vi "Goods subiv.vi"(8 "Status":T2 {"Status - camera" scale=0.0..10.0; "Status - computer" scale=0.0..10.0; "Status - TV" scale=0.0..10.0; "Status - kettle" scale=0.0..10.0; "Status -  microwave" scale=0.0..10.0; "Status - vacuum cleaner" scale=0.0..10.0; "Status - Fridge" scale=0.0..10.0; "Status - washing machine" scale=0.0..10.0}, 9 "Order":T1) -> (2 "avalibity":bool)   [LabVIEW 2020]
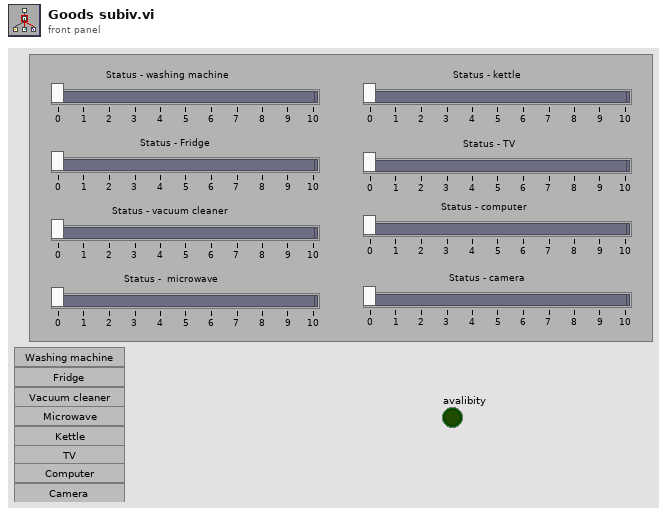
[diagram p1: front panel]
types:
  T1 = cluster{"Washing machine":bool, "Fridge":bool, "Vacuum cleaner":bool, "Microwave":bool, "Kettle":bool, "TV":bool, "Computer":bool, "Camera":bool}
  T2 = cluster{"Status - washing machine":u32, "Status - Fridge":u32, "Status - vacuum cleaner":u32, "Status -  microwave":u32, "Status - kettle":u32, "Status - TV":u32, "Status - computer":u32, "Status - camera":u32}
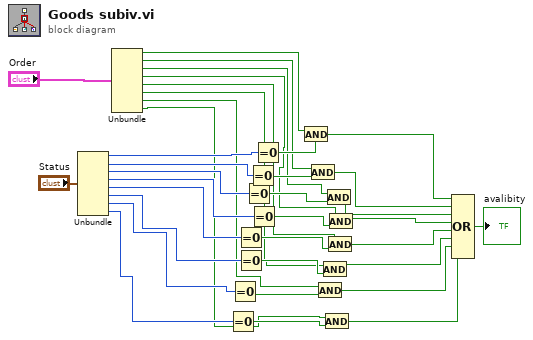
[diagram p0: block diagram]
diagram:
  n1 = Unbundle("Status") -> ("Status - washing machine"=w12:u32, "Status - Fridge"=w14:u32, "Status - vacuum cleaner"=w15:u32, "Status -  microwave"=w16:u32, "Status - kettle"=w17:u32, "Status - TV"=w18:u32, "Status - computer"=w19:u32, "Status - camera"=w20:u32)
  n2 = Unbundle("Order") -> ("Washing machine"=w9:bool, "Fridge"=w8:bool, "Vacuum cleaner"=w7:bool, "Microwave"=w6:bool, "Kettle"=w5:bool, "TV"=w4:bool, "Computer"=w3:bool, "Camera"=w2:bool)
  n3 = Equal To 0?(x=w20) -> (x = 0?=w27:bool)
  n4 = Equal To 0?(x=w19) -> (x = 0?=w26:bool)
  n5 = Equal To 0?(x=w17) -> (x = 0?=w24:bool)
  n6 = Equal To 0?(x=w18) -> (x = 0?=w25:bool)
  n7 = Equal To 0?(x=w15) -> (x = 0?=w22:bool)
  n8 = Equal To 0?(x=w14) -> (x = 0?=w21:bool)
  n9 = Equal To 0?(x=w16) -> (x = 0?=w23:bool)
  n10 = Equal To 0?(x=w12) -> (x = 0?=w13:bool)
  n11 = And(x=w9, y=w13) -> (x .and. y?=w28:bool)
  n12 = And(x=w8, y=w21) -> (x .and. y?=w29:bool)
  n13 = And(x=w3, y=w26) -> (x .and. y?=w34:bool)
  n14 = And(x=w4, y=w25) -> (x .and. y?=w33:bool)
  n15 = And(x=w2, y=w27) -> (x .and. y?=w35:bool)
  n16 = And(x=w7, y=w22) -> (x .and. y?=w30:bool)
  n17 = And(x=w5, y=w24) -> (x .and. y?=w32:bool)
  n18 = And(x=w6, y=w23) -> (x .and. y?=w31:bool)
  n19 = Compound Arithmetic op=OR(w28, w29, w30, w31, w32, w33, w34, w35) -> (→"avalibity":bool)
